vi "Get Control Refs.vi"(8 "error in (no error)":errorcluster, 11 "GaugeIndicator in":refnum<class "GaugeIndicator.lvclass">) -> (0 "error out":errorcluster, 3 "GaugeIndicator out":refnum<class "GaugeIndicator.lvclass">)   [LabVIEW 2020, in "VolatusGUIElements.lvlib" / "GaugeIndicator.lvclass"]
uses:
  GaugeIndicator.lvclass
  C:/dev/lv20CE/relink/lv-volatus/VolatusGUI/GUI Element/GUI Element.lvclass
  VolatusGUI/GUI Element/GUI Element.lvclass/GUI Element.ctl
  GaugeIndicator.lvclass/GaugeIndicator.ctl
  VolatusGUI/GUI Element/GUI Element.lvclass
  C:/dev/lv20CE/relink/lv-volatus/VolatusGUIElements/GaugeIndicator/GaugeIndicator.lvclass
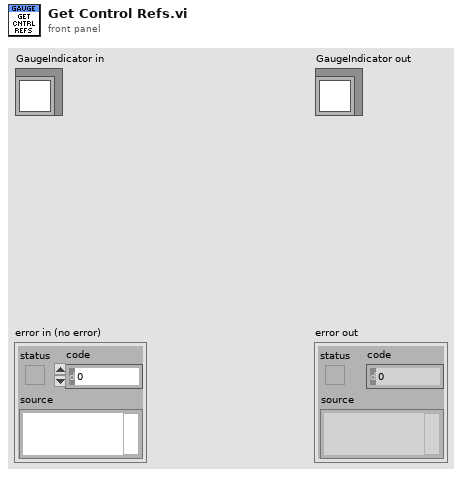
[diagram p1: front panel]
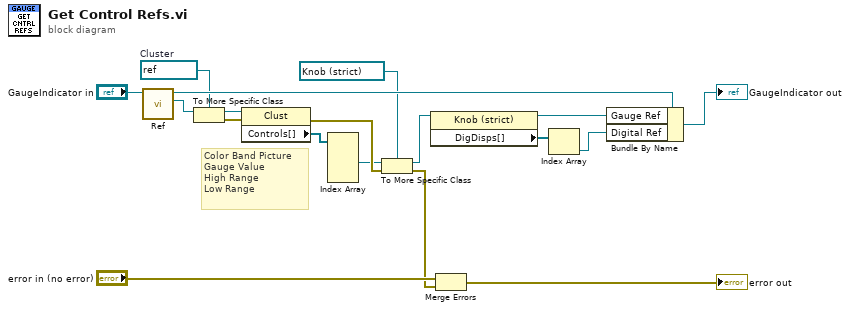
[diagram p0: block diagram]
diagram:
  w13 = refnum<vi> refnum  # Cluster
  # "Color Band Picture\nGauge Value\nHigh Range\nLow Range"
  n1 = call "Ref.vi"("GUI Element in"="GaugeIndicator in") -> ("Ref"=w14:refnum<vi>, "GUI Element out"=w15:refnum<class "GaugeIndicator.lvclass">)  [unwired: 9 in]
  n2 = To More Specific Class(target class=w13, reference=w14) -> (specific class reference=w12:refnum<vi>, error out=w11:errorcluster)  [unwired: 1 in]
  n3 = property class="Clust"(reference=w12, error in=w11) -> (error out=w18:errorcluster, "Controls[]"=w10:refnum<vi>[])  [unwired: 1 out]
  n4 = Index Array(array=w10) -> (element #2=w9:refnum<vi>)  [unwired: 4 in, 3 out]
  n5 = To More Specific Class(target class=refnum<vi> refnum ("Gauge"), reference=w9, error in=w18) -> (specific class reference=w3:refnum<vi>, error out=w5:errorcluster)
  n6 = property class="Knob (strict)"(reference=w3) -> (reference out=w1:refnum<vi>, "DigDisps[]"=w4:refnum<vi>[])  [unwired: 1 in, 1 out]
  n7 = Merge Errors("error in (no error)", w5) -> (→"error out":errorcluster)
  n8 = Index Array(array=w4) -> (element=w2:refnum<vi>)  [unwired: 1 in]
  n9 = Bundle By Name(cluster=w15, "Gauge Ref"=w1, "Digital Ref"=w2) -> (→"GaugeIndicator out":refnum<class "GaugeIndicator.lvclass">)
